vi "PH_SRDG645.PC Set Trigger.vi"(0 "i ref in":refnum<vi>, 2 "Trigger Settings":T1={"Source"=0, "Rate [Hz]"=1000.0, "Level [V]"=1.0} {"Rate [Hz]" format="%#_9p"; "Source" items=["Internal", "External rising edge", "External falling edge", "Single shot external rising edges", "Single shot external falling edges", "Single shot", "Line"]}, 5 "error IO":errorcluster) -> (14 "i ref out":refnum<vi>, 16 "something changed?":bool, 19 "error out":errorcluster)   [LabVIEW 2014, in "PH_SRDG645.lvlib"]
doc: "This VI communicates with the hardware to set the trigger settings."
uses:
  PH_SRDG645.lvlib
  PH_SRDG645.Trigger.ctl
  instr.lib/SRDG645/Stanford Research DG645 - Driver.lvlib
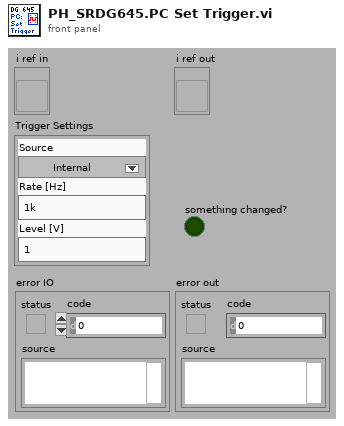
[diagram p1: front panel]
types:
  T1 = typedef "PH_SRDG645.lvlib/PH_SRDG645.Trigger.ctl" = cluster{"Source":i32, "Rate [Hz]":dbl, "Level [V]":dbl}
  T2 = typedef "PH_SRDG645.lvlib/PH_SRDG645.i attribute.ctl" = cluster{"GUI Refs":cluster{"Delete":refnum<vi>, "Device Errors":refnum<vi>, "Trigger":refnum<vi>, "Default Name":refnum<vi>, "Firmware Revision":refnum<vi>, "Serial Number":refnum<vi>, "Model":refnum<vi>, "Visa resource name":refnum<vi>}, "Service ID Rate":i32, "Service IDs Channelinfo":i32[], "VISA resource name":refnum<visa-resource-name>, "Device Errors":cluster{"code":i32, "Text":string}[], "Trigger":T1, "Channels":cluster{"T1":T3, "A":T3, "B":T3, "C":T3, "D":T3, "E":T3, "F":T3, "G":T3, "H":T3}, "GUI Refs Channels":refnum<vi>[], "Outputs":cluster{"AB":cluster{"Level Offset [V]":dbl, "Amplitue [V]":dbl, "Polarity":i32}, "CD":cluster{"Level Offset [V]":dbl, "Amplitue [V]":dbl, "Polarity":i32}, "EF":cluster{"Level Offset [V]":dbl, "Amplitue [V]":dbl, "Polarity":i32}, "GH":cluster{"Level Offset [V]":dbl, "Amplitue [V]":dbl, "Polarity":i32}, "T0":cluster{"Level Offset [V]":dbl, "Amplitue [V]":dbl, "Polarity":i32}}, "GUI Refs Outputs":refnum<vi>[], "Serial Number":string, "Firmweare Revision":string, "Model":string}
  T3 = typedef "PH_SRDG645.lvlib/PH_SRDG645.Channel Settings.ctl" = cluster{"Delay [s]":dbl, "relative to":i32}
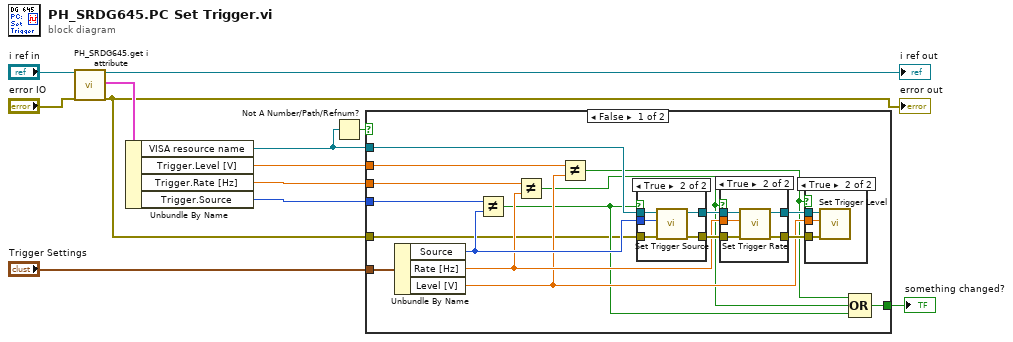
[diagram p0: block diagram]
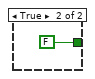
[diagram p5: hidden frame]
diagram:
  n1 = call "PH_SRDG645.get i attribute.vi"("i ref in"="i ref in", "error in (no error)"="error IO") -> ("i ref out"=→"i ref out":refnum<vi>, "i attribute"=w12:T2, "error out"=w1:errorcluster)  [unwired: 15 in]
  "error out" <- w1
  n2 = Unbundle By Name(w12) -> ("VISA resource name"=w2:refnum<visa-resource-name>, "Trigger.Level [V]"=w5:dbl, "Trigger.Rate [Hz]"=w6:dbl, "Trigger.Source"=w7:i32)
  n3 = Not A Number/Path/Refnum?(number/path/refnum=w2) -> (NaN/Path/Refnum?=w3:bool)
  n4 = case shown="False" w3 {
    tunnel: "Trigger Settings" -> [w29 _]
    tunnel: w2 -> [w28 _]
    tunnel: w7 -> [w22 _]
    tunnel: w6 -> [w21 _]
    tunnel: w5 -> [w19 _]
    tunnel: [w14 FALSE] -> w4
    tunnel: w1 -> [w13 _]
    frame False {
      n5 = Unbundle By Name(w29) -> ("Source"=w23:i32, "Rate [Hz]"=w20:dbl, "Level [V]"=w18:dbl)
      n6 = Not Equal?(x=w22, y=w23) -> (x != y?=w17:bool)
      n7 = Not Equal?(x=w21, y=w20) -> (x != y?=w15:bool)
      n8 = Not Equal?(x=w19, y=w18) -> (x != y?=w16:bool)
      n9 = case shown="True" w17 {
        tunnel: w23 -> [_ w46]
        tunnel: w28 -> [w41 w45]
        tunnel: [w40 w44] -> w27
        tunnel: w13 -> [w40 w43]
        tunnel: [w41 w42] -> w25
        frame False {
        }
        frame True {
          n10 = call "Set Trigger Source.vi"("error in (no error)"=w43, "Trigger Source (Internal)"=w46, "VISA resource name"=w45) -> ("error out"=w44:errorcluster, "VISA resource name out"=w42:refnum<visa-resource-name>)  [unwired: 6 in, 1 out]
        }
      }
      n11 = case shown="True" w15 {
        tunnel: w27 -> [w33 w39]
        tunnel: [w33 w38] -> w26
        tunnel: w20 -> [_ w37]
        tunnel: w25 -> [w34 w36]
        tunnel: [w34 w35] -> w24
        frame False {
        }
        frame True {
          n12 = call "Set Trigger Rate.vi"("error in (no error)"=w39, "Trigger Rate (1e3) [Hz]"=w37, "VISA resource name"=w36) -> ("error out"=w38:errorcluster, "VISA resource name out"=w35:refnum<visa-resource-name>)  [unwired: 6 in, 1 out]
        }
      }
      n13 = case shown="True" w16 {
        tunnel: w26 -> [_ w32]
        tunnel: w18 -> [_ w31]
        tunnel: w24 -> [_ w30]
        frame False {
        }
        frame True {
          n14 = call "Set Trigger Level.vi"("error in (no error)"=w32, "Trigger Level (1) [V]"=w31, "VISA resource name"=w30) -> ()  [unwired: 6 in, 3 out]
        }
      }
      n15 = Compound Arithmetic op=OR(w16, w15, w17) -> (w14:bool)
    }
    frame True {
    }
  }
  "something changed?" <- w4
